vi "Convert to RPM_FPGA.vi"(10 "pulses/revolution":sgl=2.0, 11 "Tach Period (uSec/pulse)":sgl) -> (3 "Tach RPM":sgl)   [LabVIEW 2014, in "Tachometer (SGL).lvlib"]
uses:
  Tachometer (SGL).lvlib
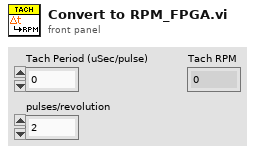
[diagram p1: front panel]
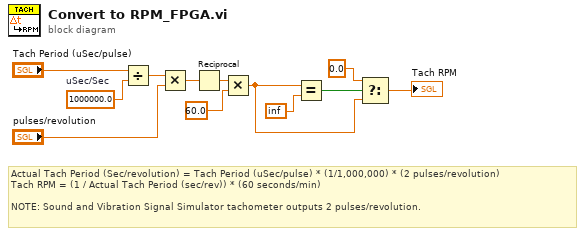
[diagram p0: block diagram]
diagram:
  w7 = sgl 1000000.0  # uSec/Sec
  # "Actual Tach Period (Sec/revolution) = Tach Period (uSec/pulse) * (1/1,000,000) * (2 pulses/revolution)\nTach RPM = (1 / Actual Tach Period (sec/rev)) * (60 seconds/min)\n\nNOTE: Sound and Vibration Signal Simulator tachometer outputs 2 pulses/revolution."
  n1 = Divide(x="Tach Period (uSec/pulse)", y=w7) -> (x/y=w9:sgl)
  n2 = Multiply(x=w9, y="pulses/revolution") -> (x*y=w8:sgl)
  n3 = Reciprocal(x=w8) -> (1/x=w11:sgl)
  n4 = Multiply(x=w11, y=sgl 60.0) -> (x*y=w2:sgl)
  n5 = Equal?(x=w2, y=sgl inf) -> (x = y?=w4:bool)
  n6 = Select(t=sgl 0.0, s=w4, f=w2) -> (s? t:f=→"Tach RPM":sgl)
